vi "Wait_ms_Example.vi"() -> ()   [LabVIEW 2017]
panel:
  in  "stop":bool
  out "Waveform Chart":dbl(graph)
  # "Objective: Generating random number(0-1) on a waveform chart every 500 ms. ."
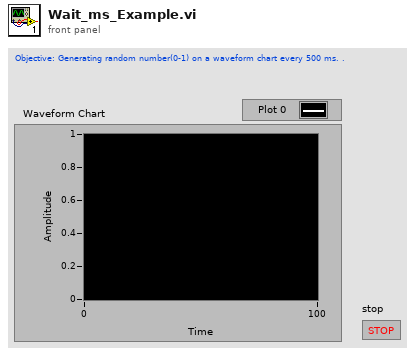
[diagram p1: front panel]
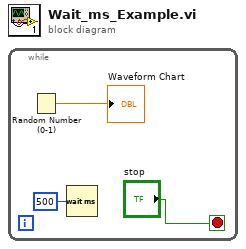
[diagram p0: block diagram]
diagram:
  n1 = while {
    stop <- "stop" stop-if-true
    n2 = Random Number (0-1)() -> (number: 0 to 1=→"Waveform Chart":dbl)
    n3 = Wait (ms)(milliseconds to wait=u32 500) -> ()  [unwired: 1 out]
  }
